vi "Begin Map.vi"   [LabVIEW 2017, in "LabPack.lvlib" / "Writer.lvclass"]
uses:
  Writer.lvclass
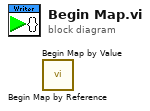
[diagram p0: block diagram]
diagram:
  n1 = call "Begin Map by Reference.vi"() -> ()  [unwired: 10 in, 2 out]
  n2 = call "Begin Map by Value.vi"() -> ()  [unwired: 10 in, 2 out]
